vi "ShooterAngleChoose.vi"(9 "Feeding Button":bool, 10 "Far 3pt Buton":bool, 11 "Close 3pt Button":bool) -> (3 "Target Shooter Angle":T1(ring))   [LabVIEW 2012]
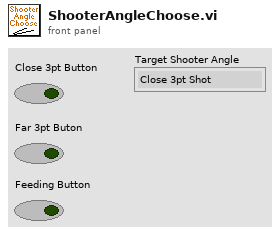
[diagram p1: front panel]
types:
  T1 = enum16{"Close 3pt Shot", "Far 3pt Shot", "Feeding"}
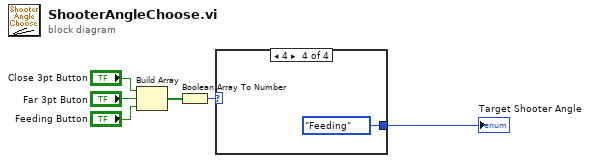
[diagram p0: block diagram]
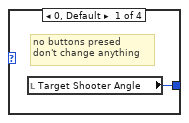
[diagram p2: hidden frame]
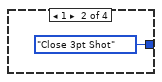
[diagram p3: hidden frame]
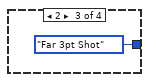
[diagram p4: hidden frame]
diagram:
  n1 = Build Array("Close 3pt Button", "Far 3pt Buton", "Feeding Button") -> (w3:bool[])
  n2 = Boolean Array To Number(Boolean array=w3) -> (number=w2:u32)
  n3 = case shown="4" w2 {
    tunnel: [w7 T1."Close 3pt Shot" ("Target Shooter Angle") T1."Far 3pt Shot" ("Target Shooter Angle") T1."Feeding" ("Target Shooter Angle")] -> w1
    frame 0, Default {
      # "no buttons presed\ndon't change anything"
      n4 = local read "Target Shooter Angle"() -> (w7:T1)
    }
    frame 1 {
    }
    frame 2 {
    }
    frame 4 {
    }
  }
  "Target Shooter Angle" <- w1
